vi "Create_Colored_Boolean_Constant.vi"() -> ()   [LabVIEW 2012]
uses:
  <vilib>/Utility/miscctls.llb/LVPointTypeDef.ctl
panel:
  in  "Colors [1]":cluster{"FG Color":u32, "BG Color":u32}[](array[cluster])=[{"FG Color"=42620, "BG Color"=10354663}]
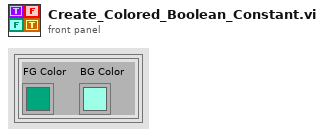
[diagram p1: front panel]
types:
  T1 = typedef "LVPointTypeDef.ctl" = cluster{"Horizontal":i16, "Vertical":i16}
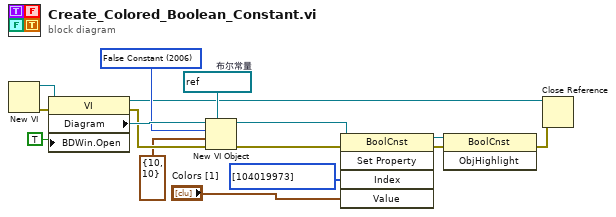
[diagram p0: block diagram]
diagram:
  w5 = u32[] [104019973] items=["Abort Callback"=104256525, "Active Bus"=518639625, "Active Cell:Active Cell"=104038415, "Active Cell:Active Cell"=416911374, "Active Cell:Active Cell"=1955905554, "Active Cell:Active Column Number"=1969896467, "Active Cell:Background Color"=1969896468, "Active Cell:Cell Background Color"=104038417, "Active Cell:Cell Background Color"=416911376, "Active Cell:Cell Background Color"=1955905556, "Active Cell:Cell Font"=104038438, "Active Cell:Cell Font"=416911397, "Active Cell:Cell Font"=1969896500, "Active Cell:Cell Font:Bold"=104038441, "Active Cell:Cell Font:Bold"=416911400, "Active Cell:Cell Font:Bold"=1969896503, "Active Cell:Cell Font:Color"=104038445, "Active Cell:Cell Font:Color"=416911404, "Active Cell:Cell Font:Color"=1969896507, "Active Cell:Cell Font:Italic"=104038442, "Active Cell:Cell Font:Italic"=416911401, "Active Cell:Cell Font:Italic"=1969896504, "Active Cell:Cell Font:Name"=104038439, "Active Cell:Cell Font:Name"=416911398, "Active Cell:Cell Font:Name"=1969896501, "Active Cell:Cell Font:Size"=104038440, "Active Cell:Cell Font:Size"=416911399, "Active Cell:Cell Font:Size"=1969896502, "Active Cell:Cell Font:Strikeout"=104038444, "Active Cell:Cell Font:Strikeout"=416911403, "Active Cell:Cell Font:Strikeout"=1969896506, "Active Cell:Cell Font:Underline"=104038443, "Active Cell:Cell Font:Underline"=416911402, "Active Cell:Cell Font:Underline"=1969896505, "Active Cell:Cell Foreground Color"=1955905555, "Active Cell:Cell Justification"=104038446, "Active Cell:Cell Justification"=416911405, "Active Cell:Foreground Color"=1969896469, "Active Cell:Cell Justification"=1969896508, "Active Cell:Cell Position"=1955905564, "Active Cell:Cell Position:Left"=1955905565, "Active Cell:Cell Position:Top"=1955905566, "Active Cell:Cell Size"=104038418, "Active Cell:Cell Size"=416911377, "Active Cell:Cell Size"=1969896470, "Active Cell:Cell Size:Height"=104038420, "Active Cell:Cell Size:Height"=416911379, "Active Cell:Cell Size:Height"=1969896471, "Active Cell:Cell Size:Width"=104038419, "Active Cell:Cell Size:Width"=416911378, "Active Cell:Cell Size:Width"=1969896472, "Active Cell:Old Cell Size"=1969896485, "Active Cell:OldHeight"=1969896486, "Active Cell:OldWidth"=1969896487, "Active Cell:Position"=104038435, "Active Cell:Position"=416911394, "Active Cell:Position"=1969896497, "Active Cell:Position:Left"=104038436, "Active Cell:Position:Left"=416911395, "Active Cell:Position:Left"=1969896498, "Active Cell:Position:Top"=104038437, "Active Cell:Position:Top"=416911396, "Active Cell:Position:Top"=1969896499, "Active Cell:String"=1969896473, "Active Cursor"=104084485, "Active Cursor"=104090629, "Active Cursor"=960400388, "Active Frame"=1721492482, "Active Item:Child-Only?"=1969896464, "Active Item:Disabled?"=1969896463, "Active Item:Indent Level"=1969896465, "Active Item:Open?"=1969896462, "Active Item:Row Number"=1969896514, "Active Item:Symbol Index"=1969896466, "Active Item:Tag"=1969896461, "Active Plot"=104081412, "Active Plot"=104084483, "Active Plot"=960400386, "Active Plot Area"=960400400, "Active Row:Active Row Number"=104035369, "Active Row:Active Row Position"=104035371, "Active Row:Active Row Position:Left"=104035372, "Active Row:Active Row Position:Top"=104035373, "Active Row:Cell Background Color"=104035374, "Active Row:Cell Font"=104035350, "Active Row:Cell Font:Bold"=104035353, "Active Row:Cell Font:Color"=104035357, "Active Row:Cell Font:Italic"=104035354, "Active Row:Cell Font:Name"=104035351, "Active Row:Cell Font:Size"=104035352, "Active Row:Cell Font:Strikeout"=104035356, "Active Row:Cell Font:Underline"=104035355, "Active Row:Cell Height"=104035370, "Active Row:Cell Justification"=104035358, "Active Slider"=104069123, "Active X Scale"=104078352, "Active Y Scale"=104078353, "Adapt To Entered Data"=98368525, "Adapt To Source"=104050718, "additionalSimulationPrivateData"=126922754, "All Objects []"=104290308, "All Objects[]"=104102916, "All Objects[]"=104105987, "All Supported Methods"=104268801, "All Supported Methods"=104268813, "All Supported Properties"=104265729, "All Supported Properties"=104265742, "All Tags"=1969896515, "Allow Absolute?"=1440002061, "Allow Create New"=49544202, "Allow Create New"=2026532874, "Allow Direct?"=1440002062, "Allow Drag"=103989253, "Allow Dragging"=104093715, "Allow Dragging (Deprecated)"=104035359, "Allow Dropping"=104032277, "Allow Dropping"=104093716, "Allow Editing Cells"=104035360, "Allow Editing Cells"=416911407, "Allow Editing Cells"=1969896509, "Allow Mixed"=867147777, "Allow Multiple Colors"=618574860, "Allow Multiple Names"=49544192, "Allow Multiple Names"=2026532864, "Allow Multiple Names"=3614191617, "Allow Multiple Rows"=618574850, "Allow No Selection"=1475095552, "Allow Preallocation"=104256517, "Allow Read?"=1440002058, "Allow Relative?"=1440002060, "Allow Scanned?"=1440002063, "Allow Selection of Parent Items"=1969896478, "Allow Transparent"=104016900, "Allow Undef Values?"=104130564, "Allow Undefined Names"=49544193, "Allow Undefined Names"=2026532865, "Allow Undefined Names"=3614191616, "Allow Undefined Names"=3813978112, "Allow Undefined Names"=3866933248, "Allow Undefined Strings"=104099842, "Allow Undefined Values"=104062976, "Allow Unwired Left Terminal"=104250373, "Allow User to Open Diagram"=1918386184, "Allow Write?"=1440002059, "AllowCreateNew"=104096791, "AllowCreateNew"=2089216013, "AllowMultiple"=104096780, "AllowMultiple"=2089216008, "AllowObjectDragAndDrop"=1918386190, "AllowRTEdits"=1918386187, "AllowUndefined"=104096779, "AllowUndefined"=2089216007, "Analog Trigger:Show AI Channels"=49544210, "Analog Trigger:Show AI Channels"=2026532882, "Analog Trigger:Show Dedicated"=49544209, "Analog Trigger:Show Dedicated"=2026532881, "Annotation List"=104084508, "Annotation List"=104090638, "Annotation List"=960400402, "Old Annotation List"=104084505, "Old Annotation List"=104090636, "Old Annotation List"=960400391, "Any Thread?"=104256515, "Array Element"=104041479, "Array Input Terminal"=104244227, "Auto Grow?"=618574861, "Auto Sizing"=104102920, "Auto Sizing Style"=104139778, "Auto Sizing?"=104139776, "Automatic Projection Mode"=1358066693, "Autoscale Delay"=104078362, "AutoSize To Fit Contents?"=104204288, "AutoSize To Fit Contents?"=897104897, "Autosizing Row Height"=104035368, "Autosizing Row Height"=104038422, "Autosizing Row Height"=416911381, "Autosizing Row Height"=1969896454, "Auto-Update From Typedef"=104013852, "Auto-Update From Typedef"=104115207, "Available Elements[]"=104250370, "Available Elements[]"=2129913858, "Background Color"=1358066689, "Bad Sub VI Linkage"=104195083, "Bar Plot Style"=103986183, "Basic Object Flags"=103983116, "Bit Accurate Data Size"=104013853, "Blinking"=104013827, "Boolean Text"=104019974, "Bounds"=103983107, "Bounds:Area Height"=103983109, "Bounds:Area Width"=103983108, "Breakpoint Status"=104173580, "Breakpoint Status"=104290314, "Breakpoint Status"=897104905, "Breakpoint?"=104271872, "BreakPoint?"=104271879, "Breakpoint?"=104290310, "Browse Button Rect"=104032276, "Browse Button:Disabled"=104032268, "Browse Button:Visible"=104032267, "Browse Dialog Options"=104032262, "Browse Options"=104032278, "Browse Options:Button Text"=104032275, "Browse Options:Match Pattern"=104032264, "Browse Options:Pattern Label"=104032269, "Browse Options:Prompt"=104032263, "Browse Options:Selection Mode"=104032265, "Browse Options:Start Path"=104032266, "Bus"=518639628, "Bus Open"=518639627, "Button Bar Visible"=104109058, "Button Size"=104019969, "Button Size"=867147778, "Button Size:Height"=104019971, "Button Size:Height"=867147780, "Button Size:Width"=104019970, "Button Size:Width"=867147779, "C Type"=104013862, "Calling Convention"=104256514, "Camera Controller:Auto Redraw"=1358066700, "Camera Controller:Type"=1358066692, "Caption"=104013828, "Caption"=104112133, "Cartesian Lines:Visible"=766554115, "Case Insensitive Match"=104222723, "Case Sensitive Pop-up"=104099846, "Cell FG Color"=104038416, "Cell FG Color"=416911375, "Cell Font"=1955905567, "Cell Font:Bold"=1955905570, "Cell Font:Color"=1955905574, "Cell Font:Italic"=1955905571, "Cell Font:Name"=1955905568, "Cell Font:Size"=1955905569, "Cell Font:Strikeout"=1955905573, "Cell Font:Underline"=1955905572, "Channel:Signal Type"=49544207, "Channel:Signal Type"=2026532879, "Chunk Size Tunnel"=104210440, "Class"=104262656, "Class ID"=103970816, "Class Name"=103970819, "Class Name"=1450114050, "Clump Num"=104173572, "Cluster Size"=104102917, "Cluster Size"=104231936, "Cluster Size:Height"=104102919, "Cluster Size:Width"=104102918, "Code Resource Path"=104253440, "CodeGenMask"=862772224, "Coerce Maximum Value"=1727315973, "Coerce Minimum Value"=1727315972, "Coercion Dot?"=104112134, "Color"=104102913, "Color"=104105984, "Color"=104290304, "Color Area Size"=104016897, "Color Area Size"=104066049, "Color Area Size:Height"=104016899, "Color Area Size:Height"=104066051, "Color Area Size:Width"=104016898, "Color Area Size:Width"=104066050, "Color Table"=104087556, "Color Table"=104090628, "Colors"=103992323, "Colors"=402934794, "Colors"=618574857, "Colors"=2056308738, "Colors [2]"=823938053, "Colors [4]"=104019973, "Colors:BG Color"=103992325, "Colors:BG Color"=402934796, "Colors:BG Color"=618574859, "Colors:BG Color"=2056308740, "Colors:FG Color"=103992324, "Colors:FG Color"=402934795, "Colors:FG Color"=618574858, "Colors:FG Color"=2056308739, "Column Header String"=104035364, "Column Header Strings[]"=104038414, "Column Header Strings[]"=416911365, "Column Header Strings[]"=1969896448, "Companion Diagram"=862772225, "Compare Aggregates?"=104179712, "Concatenate Inputs"=104247296, "Conditions"=1721492481, "Configuration Node"=1817132032, "ConfigurationNode"=1526526976, "Connected Wire"=104112128, "Constructor Node Class Name"=1777212416, "Container Bounds"=104047616, "Container Bounds"=1918386179, "Container Bounds:Height"=104047618, "Container Bounds:Height"=1918386181, "Container Bounds:Width"=104047617, "Container Bounds:Width"=1918386180, "Content Bounds"=1358066694, "Content Bounds:Height"=1358066696, "Content Bounds:Width"=1358066695, "Content Position"=1358066697, "Content Position:Horizontal"=1358066698, "Content Position:Vertical"=1358066699, "Content Rect"=104204293, "Content Rect Bounds"=104035347, "Content Rect Bounds"=104038432, "Content Rect Bounds"=416911391, "Content Rect Bounds"=1955905561, "Content Rect Bounds"=1969896494, "Content Rect Bounds:Height"=104035349, "Content Rect Bounds:Height"=104038434, "Content Rect Bounds:Height"=416911393, "Content Rect Bounds:Height"=1955905563, "Content Rect Bounds:Height"=1969896496, "Content Rect Bounds:Width"=104035348, "Content Rect Bounds:Width"=104038433, "Content Rect Bounds:Width"=416911392, "Content Rect Bounds:Width"=1955905562, "Content Rect Bounds:Width"=1969896495, "Content Rect Position"=104035344, "Content Rect Position"=104038429, "Content Rect Position"=416911388, "Content Rect Position"=1955905558, "Content Rect Position"=1969896491, "Content Rect Position:Left"=104035345, "Content Rect Position:Left"=104038430, "Content Rect Position:Left"=416911389, "Content Rect Position:Left"=1955905559, "Content Rect Position:Left"=1969896492, "Content Rect Position:Top"=104035346, "Content Rect Position:Top"=104038431, "Content Rect Position:Top"=416911390, "Content Rect Position:Top"=1955905560, "Content Rect Position:Top"=1969896493, "Content Rects[]"=897104898, "Control"=104148992, "Control"=104158211, "Control Name"=104155138, "Control Name"=104158208, "Control Reference Linked To"=59413504, "Control Reference Nodes[]"=104013833, "Control Verbs"=104047619, "Controls on Page[]"=402934786, "Controls[]"=104102914, "Controls[]"=104105985, "Convert 4.x data?"=104182784, "Convert 4.x data?"=104185856, "Convert 4.x data?"=104188928, "Cursor"=104044549, "Cursor"=104084486, "Cursor"=104090630, "Cursor"=960400389, "Cursor Color"=103989249, "Cursor Index"=103989256, "Cursor Info"=103989261, "Cursor Legend Visible"=104084496, "Cursor Legend Visible"=104090634, "Cursor Legend Visible"=960400393, "Cursor List"=104084487, "Cursor List"=104084507, "Cursor List"=104090631, "Cursor List"=104090639, "Cursor List"=960400401, "Old Cursor List"=104084506, "Old Cursor List"=104090637, "Old Cursor List"=960400390, "Cursor Lock Style"=103989254, "Cursor Name"=103989248, "Cursor Name Visible"=103989252, "Cursor Plot"=103989255, "Cursor Point Style"=103989251, "Cursor Position"=103989257, "Cursor Position:Cursor X"=103989258, "Cursor Position:Cursor Y"=103989259, "Cursor Style"=103989250, "Custom Rule"=1440002051, "Darken Compare Data"=518639616, "Data Binding:Binding Type"=104013869, "Data Binding:Blink On Alarm"=104013870, "Data Binding:LED Visible"=104013867, "Data Binding:Mode"=104013865, "Data Binding:Path"=104013864, "Data Binding:Persist ID"=104013868, "Data Binding:Status"=104013866, "Data Entry Limits"=46639105, "Data Entry Limits"=104050692, "Data Entry Limits:Increment"=46639108, "Data Entry Limits:Increment"=104050695, "Data Entry Limits:Maximum"=46639107, "Data Entry Limits:Maximum"=104050694, "Data Entry Limits:Minimum"=46639106, "Data Entry Limits:Minimum"=104050693, "Data Offset"=104271881, "DataSocket:Enabled"=104013847, "DataSocket:LED Visible"=104013854, "DataSocket:Mode"=104013846, "DataSocket:Status"=104013848, "DataSocket:URL"=104013845, "Decal Scaling?"=104019980, "DecomposerList[]"=1703848960, "Decorations"=104105986, "Decorations"=104290307, "Decorations on Page[]"=402934787, "Decorations[]"=104102915, "Decrement Key Binding"=104050705, "Default Case"=104222721, "Default Frame"=1721492480, "Default Value"=104013838, "Default Value"=104016901, "Default Value"=104032257, "Default Value"=104038421, "Default Value"=104044548, "Default Value"=104093705, "Default Value"=104096784, "Default Value"=104099841, "Default Value"=1955905537, "Default Value"=3614191619, "Default Value"=3813978114, "Default Value"=3866933250, "Defer Diagram Updates"=104109062, "Defer Panel Updates"=104105989, "Delay"=2005849094, "Deprecated_Flags"=104268806, "Deprecated_Flags[]"=104265735, "Description"=104013839, "Description"=104115201, "Description"=104173570, "Description"=104271874, "Description"=402934791, "Description"=897104900, "Device"=49544199, "Device"=2026532871, "Device String"=104096774, "Device String"=2089216002, "Diagram"=104112130, "Diagram"=104207361, "Diagram Inserted"=1918386189, "Diagrams[]"=104204291, "Diagrams[]"=897104896, "Digital Display"=104056838, "Digital Display"=104066052, "Digital Display"=104127488, "Digital Display(s) Visible"=104081417, "Digital Display[]"=104081411, "Digital Displays[]"=104069131, "Digital Line Style"=103986192, "Digital Transition Location"=103986191, "Digital Transition Type"=103986190, "Digital Tree View"=518639623, "Dimension Sizes"=104041481, "Dimension Sizes"=104121353, "Direction"=2005849088, "Disabled"=104013825, "Disabled"=104013885, "Disabled Items"=104035339, "Disabled Items"=416911362, "Disabled Items []"=104056840, "Disconnect Implicit Enable Signal"=2005849099, "Display Format"=104053766, "Display Format"=104124417, "Display Format Visible?"=104093717, "Display Format Visible?"=104136709, "Display Format:Format"=104053767, "Display Format:Format"=104124418, "Display Format:Precision"=104053768, "Display Format:Precision"=104124419, "Display Style"=104093701, "Display Style"=104136706, "Displayed Items"=1969896476, "DisplayFilter"=104096778, "DisplayFilter"=2089216006, "Doc Max"=1727315969, "Doc Min"=1727315968, "Document Bounds"=103995410, "Document Bounds:Height"=103995412, "Document Bounds:Width"=103995411, "Double-Click"=104035336, "Drag/Drop:Allow Drag and Drop Outside Control"=104035379, "Drag/Drop:Allow Drag and Drop Outside Control"=416911418, "Drag/Drop:Allow Drag and Drop Outside Control"=1969896522, "Drag/Drop:Allow Dragging"=104035376, "Drag/Drop:Allow Dragging"=416911415, "Drag/Drop:Allow Dragging"=1969896518, "Drag/Drop:Allow Dragging (Deprecated)"=416911406, "Drag/Drop:Allow Dragging (Deprecated)"=1969896483, "Drag/Drop:Allow Dragging of Parent Items"=1969896479, "Drag/Drop:Allow Dropping"=104035377, "Drag/Drop:Allow Dropping"=416911416, "Drag/Drop:Allow Dropping"=1969896519, "Drag/Drop:Allow Dropping Between Items"=1969896480, "Drag/Drop:Drag Mode"=104035378, "Drag/Drop:Drag Mode"=416911417, "Drag/Drop:Drag Mode"=1969896521, "Draw Area Size"=104044545, "Draw Companion Diagram Mask"=862772226, "DropDownList[]"=104096781, "DropDownList[]"=2089216009, "Dynamic Library?"=104256522, "Dynamic Parallel Instances Tunnel"=104210438, "Edit Position"=104038409, "Edit Position"=104038449, "Edit Position"=416911420, "Edit Position"=1955905575, "Edit Position"=1969896524, "Old Edit Position"=416911408, "Old Edit Position"=1955905547, "Old Edit Position"=1969896510, "Edit Row"=104035381, "Old Edit Row"=104035361, "Editable"=104001548, "Element"=104026112, "Element"=104121352, "Element Gap?"=104121345, "Element Names[]"=104250368, "Element Names[]"=2129913856, "Elements[]"=104139777, "Embedded Flat Sequence"=1817132036, "Enable Terminal Shown"=2005849095, "Enable Wrapping"=104093714, "Erase First"=104044546, "Error Checking Level"=104256526, "Execution Highlighted Object"=104109060, "Expand Digital Buses"=104007691, "Expand/Contract Symbol:Show Symbol at Root"=1969896520, "Expand/Contract Symbol:Symbol Type"=1969896484, "Expose Typedefs"=919859200, "FeedthroughMap"=126922755, "Fill Color"=104072194, "Fill Style"=104072193, "Fill To"=103986184, "Fill/Point Color"=103986181, "Filter On Device"=49544194, "Filter On Device"=2026532866, "FilterCriteria"=104096793, "FilterCriteria"=2089216016, "FilterOnDevice"=104096777, "FilterOnDevice"=2089216005, "FilterOnSubTypeClass"=104096776, "FilterOnSubTypeClass"=2089216004, "FilterOnTypeClass"=104096775, "FilterOnTypeClass"=2089216003, "Fire Count"=104173574, "Firing Order"=104290312, "Fix Contents"=104204297, "Fixed Tab Dimension"=618574849, "Fixed Tab Dimension:Height"=618574856, "Fixed Tab Dimension:Width"=618574855, "Fixed-Point Overflow Status Visible?"=98368527, "Fixed-Point Overflow Status Visible?"=104050720, "Fixed-Point Representation:Actual"=98368521, "Fixed-Point Representation:Actual"=104050714, "Fixed-Point Representation:Actual:Delta"=98368524, "Fixed-Point Representation:Actual:Delta"=104050717, "Fixed-Point Representation:Actual:Range Max"=98368523, "Fixed-Point Representation:Actual:Range Max"=104050716, "Fixed-Point Representation:Actual:Range Min"=98368522, "Fixed-Point Representation:Actual:Range Min"=104050715, "Fixed-Point Representation:Bits"=98368513, "Fixed-Point Representation:Bits"=104050706, "Fixed-Point Representation:Bits:Integer Word Length"=98368516, "Fixed-Point Representation:Bits:Integer Word Length"=104050709, "Fixed-Point Representation:Bits:Signed"=98368514, "Fixed-Point Representation:Bits:Signed"=104050707, "Fixed-Point Representation:Bits:Word Length"=98368515, "Fixed-Point Representation:Bits:Word Length"=104050708, "Fixed-Point Representation:Desired"=98368517, "Fixed-Point Representation:Desired"=104050710, "Fixed-Point Representation:Desired:Delta"=98368520, "Fixed-Point Representation:Desired:Delta"=104050713, "Fixed-Point Representation:Desired:Range Max"=98368519, "Fixed-Point Representation:Desired:Range Max"=104050712, "Fixed-Point Representation:Desired:Range Min"=98368518, "Fixed-Point Representation:Desired:Range Min"=104050711, "Fixed-Point Representation:Include Overflow Status?"=98368526, "Fixed-Point Representation:Include Overflow Status?"=104050719, "Flags:Has Deprecated"=104265739, "Flags:Has Ignore Errors Inside Node"=104265744, "Flags:Has Must Run At Root Loop"=104265740, "Flags:Has Not Available In AppLibs"=104265736, "Flags:Has Private"=104265737, "Flags:Has Risky Scripting"=104265741, "Flags:Has Scripting"=104265738, "Flags:Is Deprecated"=104268810, "Flags:Is Private"=104268808, "Flags:Is Risky Scripting"=104268812, "Flags:Is Scripting"=104268809, "Flags:Must Run At Root Loop"=104268811, "Flags:Not Available In AppLibs"=104268807, "Flange 1:Depth"=823938050, "Flange 1:Width"=823938048, "Flange 2:Depth"=823938051, "Flange 2:Width"=823938049, "Flavor"=104062982, "Flavor"=104130563, "Flipped"=104001546, "Focus Key Binding"=104013840, "Font"=103995393, "Font:Bold"=103995401, "Font:Color"=103995405, "Font:Italic"=103995402, "Font:Name"=103995399, "Font:Size"=103995400, "Font:Strikeout"=103995404, "Font:Underline"=103995403, "FontType"=103995416, "Force Unicode Text"=104093706, "Format"=1955905545, "Format & Precision"=103998464, "Format & Precision"=104001537, "Format & Precision:Format"=103998465, "Format & Precision:Format"=104001538, "Format & Precision:Precision"=103998466, "Format & Precision:Precision"=104001539, "Format String"=46639104, "Format String"=103998467, "Format String"=104001558, "Format String"=104053765, "Format String"=104124422, "Format String"=104259584, "Format String"=1090016256, "Formula Expression"=104225793, "Formula Parameters[]"=104225794, "Frame Count"=104216579, "Frame Names"=104222722, "Frame Rectangle"=104204294, "Frame Selector Rect"=104216578, "Frame Size"=104204290, "Frames[]"=104216577, "Frames[]"=897104903, "Full Element Index[]"=104250372, "Full Element Index[]"=2129913860, "Full Element Names[]"=104250371, "Full Element Names[]"=2129913859, "Full Name"=890692608, "Full Names Visible?"=104250369, "Full Names Visible?"=2129913857, "Function Name"=104256513, "Functions[]"=104290305, "Genericity"=104013884, "GetVRTILOErrors"=1440002066, "Graph Flavor"=104078357, "Grayed When VI Reserved"=104096797, "Grid Colors"=104007687, "Grid Colors"=104078344, "Grid Colors:Major Color"=104007688, "Grid Colors:Minor Color"=104007689, "Grid Colors:X Color"=104078345, "Grid Colors:Y Color"=104078346, "Group Member Refs[]"=103983112, "Grouped"=103983110, "Grow Info"=104013871, "Grow Info:Can Grow Horizontally"=104013872, "Grow Info:Can Grow Vertically"=104013873, "Grow Info:Max Horizontally"=104013876, "Grow Info:Max Vertically"=104013877, "Grow Info:Min Horizontally"=104013874, "Grow Info:Min Vertically"=104013875, "Grow Terms"=104195074, "GUID"=890692609, "Has Caption"=104013858, "Has Conditional Terminal?"=104210433, "Has Side Effects?"=104176642, "Has Sub-Diagram"=890692611, "Header Appearance"=2005849097, "Hide Last Value"=104056852, "Hide Text"=46639114, "Hide Text"=104053769, "High Color"=104004610, "High Color"=104010759, "Highlight Execution?"=104109059, "Horizontal Scrollbar Visible"=104041483, "Horizontal Scrollbar Visible"=104044556, "Horizontal Scrollbar Visible"=104093713, "Horizontal Scrollbar Visible"=104121356, "Horizontal Scrollbar Visible"=104139780, "Horizontal Scrollbar Visible"=1955905542, "Housing Colors"=104069133, "Housing Colors:BG Color"=104069135, "Housing Colors:FG Color"=104069134, "Housing Length"=1727315975, "Housing Size"=104069120, "Housing Size:Height"=104069122, "Housing Size:Width"=104069121, "Icon"=104173576, "Ignore Array"=104087555, "Ignore Array"=104090627, "Ignore Attributes"=104081427, "Ignore Attributes"=104084499, "Ignore Attributes"=960400395, "Ignore Errors Inside Node?"=104265733, "Ignore FPGA Reset Method"=2005849098, "Ignore Separators"=104096798, "Ignore Separators"=2089216019, "Ignore Timestamp"=104084498, "Ignore Timestamp"=960400394, "Include Invalid Names"=49544201, "Include Invalid Names"=2026532873, "Include Lower Limit?"=8582144, "Include Upper Limit?"=8582145, "IncludeInvalid"=104096790, "IncludeInvalid"=2089216012, "Increment"=1727315970, "Increment Key Binding"=104050704, "Increment/Decrement Visible?"=104053764, "Increment/Decrement Visible?"=104056851, "Independent Label"=402934793, "Index Count"=104244224, "Index Mode"=104164352, "Index Rect"=104041484, "Index Rect"=104121357, "Index Terminals[][]"=104244225, "Index Value"=104121349, "Index Values"=104038410, "Index Values"=104041476, "Index Visible"=104041475, "Index Visible?"=104121348, "Indicator"=104013831, "Initialization Type"=2005849096, "Initializer Is On Loop"=2005849093, "Initializer Terminal"=2005849091, "Initializer's Loop"=2005849092, "Input Count"=1460327424, "Input Terminal"=2005849090, "Input Terminals"=1460327425, "Input Terminals []"=104268804, "Input Terminals []"=1777212417, "Input Terminals[]"=104253442, "Input Terminals[]"=104256520, "Input?"=104152065, "Inside Terminals[]"=104161280, "Interpolate Color"=104004608, "Interpolate Color"=104010757, "Interpret As Unicode"=103995409, "Invert Inputs?[]"=104241153, "Invoke Node Class Name"=104268802, "Invoke Nodes[]"=104013836, "IOVLocalAccessMode"=1440002064, "Is Array?"=104035365, "Is Array?"=416911411, "Is Array?"=1969896513, "Is Asynchronous"=104173575, "Is Break Point Set"=104173571, "Is Break Point Set"=897104902, "Is Broken?"=104271876, "Is Debugging Allowed"=104210439, "Is On Block Diagram?"=103970821, "Is On Connector Pane"=104013856, "Is Parallelism Enabled?"=104210436, "Is Private Class Selected"=1450114052, "Is Run At Any Loop"=104173578, "Is Scripting Class Selected"=1450114051, "Is Source?"=104112131, "Is Strict"=1280954370, "Is Strict?"=1771824128, "Is Stub?"=104013883, "Is Typedef?"=104013850, "Is Typedef?"=104115205, "Is Vertical?"=2056308736, "Is Wizard Locked"=103983117, "IsCompilation"=862772227, "IsTracking"=104019977, "Item Names"=104035337, "Item Names"=416911360, "Item Symbols"=104035338, "Item Symbols"=416911361, "Items[]"=104127489, "Joints[]"=104271877, "Justification"=103995413, "Justify Tabs"=618574851, "Key Focus"=104013826, "Keyboard Mode"=104035332, "Keyboard Mode"=416911412, "Keyboard Mode"=1969896459, "Label"=104013829, "Label"=104115202, "Label"=104148993, "Label"=104155139, "Label"=104158210, "Label"=104173569, "Label"=897104899, "Label"=2056308743, "Label Format"=103986189, "Latch Value"=104013855, "Left Data Node"=1526526981, "Left Registers[]"=104167424, "Legend:Autosize"=104081425, "Legend:Autosize"=104084500, "Legend:Disable"=104081426, "Legend:Disable"=104084501, "Legend:Disable"=960400396, "Legend:Number of Rows"=104081428, "Legend:Number of Rows"=104084510, "Legend:Plot Minimum"=104081429, "Legend:Plot Minimum"=104084509, "Legend:Plots Shown"=104081424, "Legend:Plots Shown"=104084495, "Legend:Position"=104081418, "Legend:Position"=104084489, "Legend:Position:Left"=104081419, "Legend:Position:Left"=104084490, "Legend:Position:Top"=104081420, "Legend:Position:Top"=104084491, "Legend:Scrollbar Visible"=104081430, "Legend:Scrollbar Visible"=104084511, "Legend:Size"=104081421, "Legend:Size"=104084492, "Legend:Size:Height"=104081423, "Legend:Size:Height"=104084494, "Legend:Size:Width"=104081422, "Legend:Size:Width"=104084493, "Legend:Visible"=104081409, "Legend:Visible"=104084481, "Legend:Visible"=960400384, "Library Path"=104256512, "Limit To Single Line?"=104093703, "Limit To Single Line?"=104136707, "Line Style"=103986180, "Line Style"=103989262, "Line Width"=103986182, "Line Width"=103989263, "Linked Control"=104265734, "Linked Control"=104268803, "Load and Retain"=104198146, "Local Variables[]"=104013834, "Lock"=103995415, "Lock"=104075265, "Lock Boolean Text In Center"=104019975, "Locked"=103983111, "Loop Count"=104210432, "Loop Counter"=104207360, "Loop End Ref"=104210434, "Loop End Ref"=104213504, "Loose Fit"=104007684, "Loose Fit"=104010756, "Low Color"=104004609, "Low Color"=104010758, "Mapping Mode"=104001547, "Marker"=104001557, "Marker Colors"=104001554, "Marker Colors:BG Color"=104001556, "Marker Colors:Text Color"=104001555, "Marker Values[]"=104004611, "Marker Values[]"=104007685, "Marker Values[]"=104010760, "Master Bounds Rect"=103983115, "MatchFirstInList"=104099847, "Mechanical Action"=104019976, "Mechanical Action"=1475095553, "Menu Button Visible"=104096795, "Menu Button Visible"=2089216018, "Menubar Visible"=104105993, "Menubar Visible"=104109057, "Method"=104268800, "Method"=104268814, "Minor Tick Color"=104001550, "Mode"=104241152, "ModelView Matrix"=1358066688, "Modified"=103970820, "Mouse"=104044547, "Multiple Line Input"=104035367, "Multiple Line Input"=104038424, "Multiple Line Input"=416911383, "Multiple Line Input"=1969896455, "Multiple Text String"=104019978, "Name"=104112132, "Name"=104152064, "Name Format"=104262657, "Name Label"=104007686, "Name Label"=104010762, "Named Numeric Colors"=104056835, "Named Numeric Colors:BG Color"=104056837, "Named Numeric Colors:Text Color"=104056836, "Named Numeric Font"=104056842, "Named Numeric Font:Bold"=104056845, "Named Numeric Font:Color"=104056849, "Named Numeric Font:Italic"=104056846, "Named Numeric Font:Name"=104056843, "Named Numeric Font:Size"=104056844, "Named Numeric Font:Strikeout"=104056848, "Named Numeric Font:Underline"=104056847, "Named Numeric Size"=104056832, "Named Numeric Size:Height"=104056834, "Named Numeric Size:Width"=104056833, "NI Validated"=104256518, "Nodes"=104290313, "Num Dimensions"=104121344, "Num Of Sliders"=104069128, "Number of Columns"=104038401, "Number of Columns"=104041473, "Number of Columns"=104121346, "Number of Columns"=416911370, "Number of Columns"=1969896452, "Number Of Dimensions"=104041480, "Number of Items"=104056841, "Number of Rows"=104035329, "Number of Rows"=104038402, "Number of Rows"=104041474, "Number of Rows"=104121347, "Number of Rows"=416911369, "Number of Rows"=1969896451, "Number of Static Parallel Instances"=104210437, "Numeric Text"=46639113, "Numeric Text"=104053763, "Numeric Text"=104124423, "Numeric Text"=1090016257, "Objects on Page[]"=402934788, "Offset and Multiplier"=104007681, "Offset and Multiplier"=104010753, "Offset and Multiplier:Multiplier"=104007683, "Offset and Multiplier:Multiplier"=104010755, "Offset and Multiplier:Offset"=104007682, "Offset and Multiplier:Offset"=104010754, "Old Cursor List"=104084497, "Old Format & Precision"=104050688, "Old Format & Precision:Old Format"=104050689, "Old Format & Precision:Old Precision"=104050690, "Old Format String"=104050703, "Old Out of Range Action"=104050696, "Old Range"=104001553, "Optional Plane:Labels Visible"=766554114, "Optional Plane:Lines Visible"=766554113, "Optional Plane:Plane Type"=766554112, "Origin"=104044550, "Origin"=1918386188, "Origin:Left"=104044551, "Origin:Left"=404044551, "Origin:Top"=104044552, "Output Count"=1556456448, "Output Node"=1817132033, "Output Terminal"=2005849089, "Output Terminals []"=104256519, "Output Terminals []"=104268805, "Output Terminals []"=1777212418, "Output Terminals[]"=104244228, "Output Terminals[]"=104253443, "Output Terminals[]"=1556456449, "Output Terminals[] (Deprecated)"=104244226, "OutputNode"=1526526977, "Outside Terminal"=104161281, "Owner (Deprecated)"=103970817, "Owner"=103970822, "Owning VI"=103970818, "Page Enabled State"=402934784, "Page Label"=402934790, "Page Labels Display Visible?"=618574863, "Page Selector Visible"=65605632, "Page Size"=1727315971, "Page Visible"=402934785, "Pages"=65605633, "Palette:Active Tool"=104078351, "Palette:Visible"=104078339, "Panel Transparent"=1918386178, "Panes"=104105990, "Parallel Schedule"=104210441, "Parameter Info"=104256516, "Parameter Info"=104256521, "ParameterCount"=104253441, "Path Text"=104032261, "Path Type"=104118274, "Physical Channel:Show External"=49544216, "Physical Channel:Show External"=2026532888, "Physical Channel:Show Internal"=49544217, "Physical Channel:Show Internal"=2026532889, "Physical Channel:Show Internal Bizarre"=49544218, "Physical Channel:Show Internal Bizarre"=2026532890, "Physical Channel:Signal Type"=49544208, "Physical Channel:Signal Type"=2026532880, "Pipe Radius"=823938052, "Pixel Width"=104035330, "Plot"=104081413, "Plot"=104084484, "Plot"=960400387, "Plot Area Bounds"=104078361, "Plot Area:Colors"=104078341, "Plot Area:Colors:BG Color"=104078343, "Plot Area:Colors:FG Color"=104078342, "Plot Area:Position"=104078358, "Plot Area:Position:Left"=104078359, "Plot Area:Position:Top"=104078360, "Plot Area:Size"=104078336, "Plot Area:Size:Height"=104078338, "Plot Area:Size:Width"=104078337, "Plot Color"=103986177, "Plot Images:Back"=104084502, "Plot Images:Back"=960400397, "Plot Images:Front"=104084504, "Plot Images:Front"=104090635, "Plot Images:Front"=960400399, "Plot Images:Middle"=104084503, "Plot Images:Middle"=960400398, "Plot Info"=103986188, "Plot Interpolation"=103986178, "Plot Name"=103986176, "Point Style"=103986179, "Position"=103983104, "Position:Left"=103983105, "Position:Top"=103983106, "Prealloc Length"=104093707, "Prealloc Length"=104136708, "Probe"=104271873, "ProbeVI"=104274945, "Projection Matrix"=1358066691, "Properties[]"=104265728, "Properties[]"=104265743, "Property Count"=104265731, "Property Items[]"=104265730, "Property Node Class Name"=104265732, "Property Nodes[]"=104013835, "Radix Visible?"=104053762, "Radix Visible?"=104124420, "Ramp Visible"=104004612, "Ramp Visible"=104010761, "Range"=104001540, "Range:Increment"=104001543, "Range:Maximum"=104001542, "Range:Minimum"=104001541, "Range:Minor Increment"=104001544, "Range:Start"=104001545, "Recomposer List[]"=1703848961, "Region Nodes[]"=890692610, "Relative Mode"=1440002052, "Reload For Each Call"=104198145, "Representation"=98368512, "Representation"=104050691, "Representation"=1727315974, "Reserve Callback"=104256523, "Resize Info:Can Resize Horizontally"=103983119, "Resize Info:Can Resize Vertically"=103983120, "Resize Info:Include In Resize"=103983122, "Resize Info:Name in Resize Dialog"=103983121, "Resource Id"=104176643, "Response to Value Outside Limits"=46639109, "Response to Value Outside Limits"=104050699, "Response to Value Outside Limits:Increment"=46639112, "Response to Value Outside Limits:Increment"=104050702, "Response to Value Outside Limits:Maximum"=46639110, "Response to Value Outside Limits:Maximum"=104050700, "Response to Value Outside Limits:Minimum"=46639111, "Response to Value Outside Limits:Minimum"=104050701, "RestrictLRGrowMove"=104250374, "RestrictLRGrowMove"=2129913861, "RGB Value"=104066055, "Right Data Node"=1526526982, "Right Shift Register"=104287232, "Ring Text"=104056850, "Row Header Strings[]"=104038413, "Row Header Strings[]"=416911410, "Row Header Strings[]"=1969896512, "Scale"=104066053, "Scale"=104072195, "Scale"=104075264, "Scale Fit"=104007680, "Scale Fit"=104010752, "Scale Info"=104066054, "Scale Info"=104069132, "Scale Legend:Visible"=104078354, "Scale Panel"=1918386176, "Scroll Position"=103995397, "Scrollbar Visible"=104032274, "Scrollbar Visible"=104093702, "Scrollbar Visible?"=104118273, "Scrollbar Visible?"=104136705, "Scrollbar Visible?"=104225792, "Scrollbars Visible"=104044554, "Select Entire Rows"=104035380, "Select Entire Rows"=416911419, "Select Entire Rows"=1969896523, "Selected"=103983113, "Selected Cell"=416911384, "Selected Cursors"=104084488, "Selected Cursors"=104090632, "Selected Cursors"=960400392, "Selection"=103995394, "Selection Color"=104035366, "Selection Color"=104038408, "Selection Color"=416911380, "Selection Color"=1955905550, "Selection Color"=1969896456, "Selection End[]"=104121351, "Selection List[]"=104105988, "Selection List[]"=104109056, "Selection Mode"=104035331, "Selection Mode"=416911373, "Selection Mode"=1969896460, "Selection Size"=104038412, "Selection Size"=1955905549, "Selection Size[]"=104041478, "Selection Start"=104038411, "Selection Start"=1955905548, "Selection Start[]"=104041477, "Selection Start[]"=104121350, "Selection:End"=103995396, "Selection:Start"=103995395, "SelectionModeFlags"=289982464, "Selector"=104222720, "Sequence Locals[]"=104219648, "Shared Clones:Automatic Allocation Strategy Enabled"=104204295, "Shared Clones:Pre-Allocate"=104204296, "Shared Variable Project Item"=1440002048, "Shift Registers[]"=104207362, "Short Count"=104173573, "Show Buses With Lines"=518639624, "Show Selection?"=104121354, "Show Timeout?"=1440002053, "Show Timestamp?"=1440002050, "Show Value Tip Strip"=104069136, "Sibling Multiselect"=1969896516, "Signal Numbers Visible"=1955905544, "SimDiagisDirty"=126922756, "SimulationDiagram"=1988411392, "SimulationParameters"=126922753, "Size"=103992320, "Size"=104032271, "Size"=104035341, "Size"=104038426, "Size"=104093709, "Size"=104096786, "Size"=416911385, "Size"=1955905538, "Size"=1969896488, "Size to Text?"=103995398, "Size To Text?"=104118272, "Size To Text?"=104136704, "Size:Height"=103992322, "Size:Height"=104032273, "Size:Height"=104035343, "Size:Height"=104038428, "Size:Height"=104093711, "Size:Height"=104096788, "Size:Height"=416911387, "Size:Height"=1955905540, "Size:Height"=1969896490, "Size:Width"=103992321, "Size:Width"=104032272, "Size:Width"=104035342, "Size:Width"=104038427, "Size:Width"=104093710, "Size:Width"=104096787, "Size:Width"=416911386, "Size:Width"=1955905539, "Size:Width"=1969896489, "Sizing"=2056308742, "Skip Subroutine Call If Busy"=104195077, "Skip When Tabbing"=104013857, "Slider Colors"=104069124, "Slider Colors:BG Color"=104069126, "Slider Colors:FG Color"=104069125, "Smooth Horizontal Scrolling"=104038423, "Smooth Horizontal Scrolling"=416911382, "Smooth Update"=104084482, "Smooth Update"=104090625, "Smooth Update"=960400385, "SnaptoMouse"=104075266, "Source Addressing Mode"=104271880, "Splitter Position"=2056308737, "Splitter Position Locked"=2056308741, "Splitters[]"=104105991, "Stack Plots?"=104081415, "State Nodes[]"=827376640, "Static VI Path"=104198144, "StaticState"=862772228, "Stop If True?"=104210435, "Stop If True?"=104213505, "Strings []"=104056839, "Strings []"=104099843, "Strings []"=867147776, "Strings []"=2145735680, "Strings [4]"=104019972, "Strings And Values []"=104062980, "Strings And Values []"=104099844, "Strings And Values []"=104130561, "Strings And Values []"=2145735681, "Style"=104001536, "Style"=104142848, "Style"=104173577, "Style"=104176641, "Style ID"=104013882, "SubTypeClass"=104096773, "SubTypeClass"=2089216001, "SubVI Setup:Close Front Panel After Call"=104195081, "SubVI Setup:Open Front Panel When Loaded"=104195079, "SubVI Setup:Show Front Panel When Called"=104195080, "SubVI Setup:Suspend When Called"=104195082, "SubVIs[]"=104290306, "Switch:Show Channels"=49544211, "Switch:Show Channels"=2026532883, "Switch:Show Relays"=49544212, "Switch:Show Relays"=2026532884, "Switch:Show Topologies"=49544219, "Switch:Show Topologies"=2026532891, "Synch Current And Default Values"=104096796, "Synchronous Display"=104013832, "Synchronous I/O?"=104192000, "Tab Caption"=402934789, "Tab Control Pane Dimension"=618574852, "Tab Control Pane Dimension:Height"=618574854, "Tab Control Pane Dimension:Width"=618574853, "Tab Into"=618574866, "Tab Layout"=618574864, "Tab Location"=618574865, "Tab Size"=618574848, "Tabs Visible?"=618574862, "TagList[]"=104096789, "TagList[]"=2089216011, "TagType"=49544200, "TagType"=104096783, "TagType"=2026532872, "TagType"=2089216014, "Target Syntax Checking"=104204292, "Target Syntax Checking"=897104904, "Terminal"=104013830, "Terminal"=104115204, "Terminal"=104152066, "Terminal"=1450114049, "Terminal Height"=104235008, "Terminal:Show Advanced"=49544214, "Terminal:Show Advanced"=2026532886, "Terminal:Show Basic"=49544213, "Terminal:Show Basic"=2026532885, "Terminal:Show Private"=49544215, "Terminal:Show Private"=2026532887, "Terminals Visible?"=104176640, "Terminals Visible?"=104195072, "Terminals[]"=104170496, "Terminals[]"=104173568, "Terminals[]"=104271875, "Terminals[]"=897104901, "Text"=103995392, "Text"=104093700, "Text"=104096771, "Text"=867147781, "Text Colors"=103995406, "Text Colors:BG Color"=103995408, "Text Colors:Text Color"=103995407, "Text Focus"=104105992, "Text Focus"=104109061, "Text Labels Visible?"=104069129, "Text Labels[]"=104069130, "Text Size"=104032258, "Text Size"=104093697, "Text Size"=104096768, "Text Size:Height"=104032260, "Text Size:Height"=104093699, "Text Size:Height"=104096770, "Text Size:Width"=104032259, "Text Size:Width"=104093698, "Text Size:Width"=104096769, "Text Width"=104053761, "Tick Color"=104001549, "Timed Loop Left DCO"=1526526978, "Timed Loop Right DCO"=1526526979, "Timed Sequence Left DCO"=1817132034, "Timed Sequence Right DCO"=1817132035, "Timeout Allowed?"=1440002054, "Timestamp Allowed?"=1440002065, "Tip Strip"=104013844, "Tip Strip"=104115203, "Tip Strip"=402934792, "TL Timed Sequence"=1526526980, "Toggle Key Binding"=104019979, "Toggle Key Binding"=867147782, "Top Left Cell"=1955905546, "Top Left Visible Cell"=416911372, "Top Left Visible Cell"=1969896457, "Top Row"=104035335, "Total Bounds Rect"=103983114, "Transitions Visible"=1955905543, "Transpose Array"=104078340, "Tunnel"=104284160, "Tunnels[]"=104204289, "Twisty Type"=1969896474, "Type"=1450114048, "Type Class"=1493837824, "Type Descriptor"=104013841, "Type Descriptor"=104112129, "Type Descriptor (Full)"=104013863, "TypeClass"=104096772, "TypeClass"=2089216000, "Typedef:Path"=104013851, "Typedef:Path"=104115206, "Typedef:VI"=104013861, "Typedef:VI"=104115208, "UID"=103983123, "Uniform Marker Spacing?"=104001551, "Unit"=104201216, "Unit Label"=104007690, "Unit Label"=104010763, "Unit Label"=104050698, "Unit Label"=104124424, "Unit Label Visible?"=104124421, "Unreserve Callback"=104256524, "Update Mode"=104081414, "Update Mode"=104087557, "Update While Typing?"=104093704, "UpdatedTagList[]"=104096792, "UpdatedTagList[]"=2089216015, "User Data"=104023040, "User Data"=104096794, "User Data"=1333814273, "User Data"=2089216017, "Value"=104013837, "Value"=104016896, "Value"=104032256, "Value"=104038400, "Value"=104044544, "Value"=104093696, "Value"=104096782, "Value"=104099840, "Value"=104115200, "Value"=1333814272, "Value"=1918386185, "Value"=1955905536, "Value"=2089216010, "Value"=3614191618, "Value"=3813978113, "Value"=3866933249, "Value (Signaling)"=104013859, "Value (Signaling)"=104016902, "Value (Signaling)"=104032270, "Value (Signaling)"=104038425, "Value (Signaling)"=104044555, "Value (Signaling)"=104093708, "Value (Signaling)"=104096785, "Value (Signaling)"=104099845, "Value (Signaling)"=1918386186, "Value (Signaling)"=1955905557, "Value (Signaling)"=3614191620, "Value (Signaling)"=3813978115, "Value (Signaling)"=3866933251, "Values []"=104062979, "Values []"=104130560, "Vertical Arrangement"=103995414, "Vertical Scrollbar Visible"=104041482, "Vertical Scrollbar Visible"=104044557, "Vertical Scrollbar Visible"=104093712, "Vertical Scrollbar Visible"=104121355, "Vertical Scrollbar Visible"=104139779, "Vertical Scrollbar Visible"=1955905541, "VI Name"=104155136, "VI Name"=104195073, "VI Name"=1280954368, "VI Path"=104195075, "VI Path"=1280954369, "VI Reference"=104195078, "View As Icon"=104139781, "View As Icon"=104195076, "Visible"=103986187, "Visible"=103989260, "Visible"=103992326, "Visible"=104001552, "Visible"=104013824, "Visible"=104173579, "Visible Bounds"=104290311, "Visible Frame"=104216576, "Visible Items:Column Header Visible"=104035363, "Visible Items:Column Headers Visible"=104038407, "Visible Items:Column Headers Visible"=416911371, "Visible Items:Column Headers Visible"=1969896453, "Visible Items:Hierarchy Lines Visible"=1969896525, "Visible Items:Hierarchy Lines Visible Old"=1969896477, "Visible Items:Horizontal Lines Visible"=104035375, "Visible Items:Horizontal Lines Visible"=104038447, "Visible Items:Horizontal Lines Visible"=416911414, "Visible Items:Horizontal Lines Visible"=1969896482, "Visible Items:Horizontal Scrollbar Visible"=104038405, "Visible Items:Horizontal Scrollbar Visible"=416911368, "Visible Items:Horizontal Scrollbar Visible"=1969896450, "Visible Items:Index Visible"=104038403, "Visible Items:Row Headers Visible"=104038406, "Visible Items:Row Headers Visible"=416911409, "Visible Items:Row Headers Visible"=1969896511, "Visible Items:Symbols Visible"=104035334, "Visible Items:Symbols Visible"=416911366, "Visible Items:Symbols Visible"=1969896458, "Visible Items:Vertical Lines Visible"=104038448, "Visible Items:Vertical Lines Visible"=416911413, "Visible Items:Vertical Lines Visible"=1969896481, "Visible Items:Vertical Scrollbar Visible"=104035333, "Visible Items:Vertical Scrollbar Visible"=104038404, "Visible Items:Vertical Scrollbar Visible"=416911367, "Visible Items:Vertical Scrollbar Visible"=1969896449, "Wire"=104274944, "Wire Width"=104271878, "Wires[]"=104290309, "Wizard Data"=104013849, "Write?"=104155137, "Write?"=104158209, "Write?"=1440002049, "X Scale"=104078347, "X Scale Index"=103986185, "X Scale Info"=104078349, "X Scrollbar Visible"=104078356, "X Scrollbar Visible"=1918386182, "XControl:Container Bounds"=104013879, "XControl:Container Bounds:Height"=104013881, "XControl:Container Bounds:Width"=104013880, "XControl:Is XControl?"=104013878, "Y Scale"=104078348, "Y Scale Index"=103986186, "Y Scale Info"=104078350, "Y Scrollbar Visible"=1918386183, "Z Scale"=104087554, "Z Scale"=104090626, "Z Scale Info"=104090633, "Zoom Factor"=104044553] ("Index")
  w9 = refnum<vi> refnum  # 布尔常量
  w11 = 2006 items=[".NET Container"=2125, ".NET Refnum"=3441, "2D Picture"=3508, "3D Picture"=23776, "Absolute Value"=1054, "Access Rights"=1412, "ActiveX Container"=2072, "Add"=1050, "Add (with error terminals)"=3915, "Add Array Elements"=1903, "Agitator"=3831, "AllSpoll"=1960, "Always Copy"=2400, "And"=1061, "And Array Elements"=1911, "Append True/False String"=1511, "Application Refnum"=3412, "Array (block diagram constant)"=2070, "Array (classic)"=3300, "Array (modern)"=21608, "Array Interface Control"=23777, "Array Max & Min"=1907, "Array of Strings to Path"=1422, "Array Size"=1809, "Array Subset"=2044, "Array To Cluster"=1168, "Array To Spreadsheet String"=1540, "Atmospheric Tank (classic)"=3070, "Atmospheric Tank (modern)"=21751, "Automation Close"=8001, "Automation Open"=8000, "Automation Refnum"=3410, "Avogadro Constant (1/mol)"=23520, "Base 10 Logarithm Of e"=23512, "Bin #1"=3073, "Bin #2"=21755, "Bitpack to Array"=3135, "Bluetooth Close Connection"=9148, "Bluetooth Create Listener"=9151, "Bluetooth Discover"=9152, "Bluetooth Network Connection Refnum"=3468, "Bluetooth Open Connection"=9153, "Bluetooth Read"=9149, "Bluetooth Wait On Listener"=9147, "Bluetooth Write"=9150, "Boolean Array To Number"=1815, "Boolean To (0,1)"=1167, "Build Array"=2041, "Build Cluster Array"=2047, "Build Matrix"=8500, "Build Path"=1419, "Build Waveform"=2066, "Bundle"=2049, "Bundle By Name"=2057, "Byte Array To String"=1609, "Byte Stream File Refnum"=3408, "Call By Reference"=3901, "Call Chain"=1999, "Call Library Function Node"=2062, "Call Parent Method"=2354, "CAN Channel (block diagram constant)"=2124, "CAN Channel (classic)"=3340, "CAN Channel (modern)"=21817, "CAN Channel (system)"=21966, "CAN Interface (block diagram constant)"=2123, "CAN Interface (classic)"=3339, "CAN Interface (modern)"=21815, "CAN Interface (system)"=21964, "CAN Task (block diagram constant)"=3471, "CAN Task (classic)"=3470, "CAN Task (modern)"=21789, "CAN Task (system)"=21963, "Cancel Button (modern)"=21739, "Cancel Button (system)"=3131, "Cancel Notification"=9107, "Carriage Return Constant"=23500, "Case Structure"=2001, "Cast Unit Bases"=1079, "Check Valve"=3833, "Checkbox (classic)"=3117, "CheckBox (modern)"=21924, "Checkbox (system)"=3132, "Class Specifier Constant"=2094, "Clear Fixed-Point Overflow Status"=5562, "Close File"=8052, "Close File (deprecated)"=1405, "Close Reference"=8011, "Close Variable Connection"=23783, "Cluster (classic)"=3400, "Cluster (modern)"=21607, "Cluster Constant"=2071, "Cluster To Array"=1169, "Code Interface Node"=2050, "Coerce To Type"=2402, "Color Box"=3013, "Color Box Constant"=2120, "Color Box Thin Border"=2905, "Color Ramp"=3022, "Colored Rectangle (broken?)"=3625, "Combo Box (classic)"=3304, "Combo Box (modern)"=21604, "Combo Box (system)"=21917, "Combo Box Constant"=2088, "Complex Conjugate"=1048, "Complex To Polar"=1045, "Complex To Re/Im"=1044, "Compound Arithmetic"=2200, "Compressor"=3832, "Concatenate Strings"=2040, "Conditional Disable Structure"=2064, "Constructor Node"=3904, "Control & Simulation Loop"=2099, "Control Help Window"=1353, "Control Online Help"=1355, "Control Refnum"=3419, "Convert Unit"=2059, "Conveyer"=3827, "Copy"=8053, "Copy (deprecated)"=1416, "Cosecant"=1204, "Cosine"=1201, "Cotangent"=1205, "CPU Information"=24130, "Create Folder"=8055, "Create Network Stream Reader Endpoint"=23811, "Create Network Stream Writer Endpoint"=23810, "Create Stream"=23796, "Create User Event"=2073, "Current Processor ID"=24131, "Current VI's Menubar"=9000, "Current VI's Path"=1426, "DAQmx Analog Trigger Source (block diagram constant)"=2119, "DAQmx Analog Trigger Source (classic)"=3336, "DAQmx Analog Trigger Source (modern)"=21774, "DAQmx Analog Trigger Source (system)"=21951, "DAQmx Device Name (block diagram constant)"=2093, "DAQmx Device Name (classic)"=3318, "DAQmx Device Name (modern)"=21773, "DAQmx Device Name (system)"=21950, "DAQmx Global Channel (block diagram constant)"=3430, "DAQmx Global Channel (classic)"=3443, "DAQmx Global Channel (modern)"=21770, "DAQmx Global Channel (system)"=21957, "DAQmx Physical Channel (block diagram constant)"=2118, "DAQmx Physical Channel (classic)"=3335, "DAQmx Physical Channel (modern)"=21777, "DAQmx Physical Channel (system)"=21954, "DAQmx Scale Name (block diagram constant)"=2116, "DAQmx Scale Name (classic)"=3317, "DAQmx Scale Name (modern)"=21775, "DAQmx Scale Name (system)"=21952, "DAQmx Switch (block diagram constant)"=2121, "DAQmx Switch (classic)"=3337, "DAQmx Switch (modern)"=21776, "DAQmx Switch (system)"=21953, "DAQmx Task Name (block diagram constant)"=3434, "DAQmx Task Name (classic)"=3442, "DAQmx Task Name (modern)"=21778, "DAQmx Task Name (system)"=21959, "DAQmx Terminal (block diagram constant)"=2117, "DAQmx Terminal (classic)"=3319, "DAQmx Terminal (modern)"=21781, "DAQmx Terminal (system)"=21955, "Data Cache Size"=24132, "Data Log File Refnum"=3402, "Data Value Reference"=3476, "Data Value Reference Constant"=24134, "DataSocket Close"=1085, "DataSocket Open"=1084, "DataSocket Read"=1086, "DataSocket Refnum"=3417, "DataSocket Write"=1087, "Date/Time To Seconds"=1308, "Decimal Digit?"=1119, "Decimal String To Number"=1184, "Decimate 1D Array"=2046, "DecomposeArray"=2412, "DecomposeLockDataValRef"=2406, "DecomposeVariant"=2404, "Decrement"=1058, "Default Directory"=1427, "Delete"=8056, "Delete (deprecated)"=1417, "Delete Data Value Reference"=2409, "Delete From Array"=3912, "Delete Menu Items"=9004, "Delete Variant Attribute"=8206, "Delete Waveform Attribute"=8209, "Deny Access"=8057, "Dequeue Element"=9113, "Destroy Stream Endpoint"=23794, "Destroy User Event"=2075, "DevClear"=1961, "DevClearList"=1962, "Device Control/Status"=1433, "Device Refnum"=3405, "Diagram Disable Structure"=2054, "Dial (classic)"=3050, "Dial (modern)"=21732, "Digital Data (classic)"=3210, "Digital Data (modern)"=21216, "Digital Waveform Graph (classic)"=3511, "Digital Waveform Graph (modern)"=21718, "Direct Variable Read"=23785, "Direct Variable Write"=23788, "Divide"=1053, "Divide (with error terminals)"=3918, "Dlg Horiz Scrollbar"=21905, "Dlg Numeric #1"=2100, "Dlg Numeric #2"=3006, "Dlg String"=2110, "Dlg Vert Scrollbar"=21906, "Down Arrow"=3824, "Down Bow Valve (flat)"=3707, "Down Bow Valve (outline)"=3807, "Down Bow Valve (shaded)"=21767, "Down Rect Valve (flat)"=3706, "Down Rect Valve (outline)"=3806, "Down Rect Valve (shaded)"=21766, "Down Tee (flat)"=3818, "Down Tee (shaded)"=3718, "Dynamic FPGA Interface Cast"=5690, "Elementary Charge (C)"=23517, "Empty Array?"=23063, "Empty Path Constant"=23523, "Empty String Constant"=23503, "Empty String/Path?"=1112, "Enable Menu Tracking"=9002, "EnableLocal"=1963, "EnableRemote"=1964, "End of Line Constant"=23525, "Enqueue Element"=9111, "Enqueue Element At Opposite End"=9129, "Enum (classic)"=3023, "Enum (modern)"=21605, "Enum (system)"=3062, "Enum Constant"=2090, "EOF"=1410, "Equal To 0?"=1113, "Equal?"=1102, "Error Ring Constant"=2039, "Event Callback Refnum"=3435, "Event Data Node"=2102, "Event Structure"=2052, "Exchanger"=3828, "Exclusive Or"=1063, "Exponential"=1211, "Exponential (Arg) -1"=1222, "Expression Node"=2201, "False Constant"=2006, "Feedback Node"=2353, "FieldPoint IO Point (block diagram constant)"=3440, "FieldPoint IO Point (classic)"=3439, "FieldPoint IO Point (modern)"=21784, "FIFO Refnum"=3474, "File Dialog"=8058, "File Dialog (deprecated)"=8081, "File Path Control (classic)"=3203, "File Path Control (modern)"=21730, "File Path Control (system)"=21922, "File Path Indicator (classic)"=3204, "File Path Indicator (modern)"=21731, "File/Directory Info"=8082, "File/Directory Info (deprecated)"=1413, "FindLstn"=1965, "FindRQS"=1966, "First Call?"=1083, "Fixed-Point Overflow?"=5565, "Fixed-Point to Integer Cast"=5566, "Flat Box"=3602, "Flat Circle"=3605, "Flat Down Triangle"=3623, "Flat Frame"=3608, "Flat Left Triangle"=3620, "Flat Right Triangle"=3621, "Flat Round Button"=3102, "Flat Rounded Box"=3611, "Flat Sequence Structure"=2069, "Flat Square Button"=3103, "Flat Up Triangle"=3622, "Flatten To String"=1164, "Flatten To XML"=8400, "Flattened String To Variant"=8202, "Floating Point Equal?"=23064, "Flush File"=8059, "Flush File (deprecated)"=1406, "Flush Queue"=9114, "Flush Stream"=23808, "For Loop"=2002, "Fork"=2194, "Format Date/Time String"=8100, "Format Into File"=2083, "Format Into String"=2081, "Format Value"=1512, "Formula Node"=2004, "FPGA Refnum to Session"=2322, "Fract/Exp String To Number"=1187, "Framed Color Box (classic)"=3008, "Framed Color Box (modern)"=21019, "Free Label"=2321, "Furnace"=3829, "Gauge (classic)"=3040, "Gauge (modern)"=21009, "Gauge for Simon"=32600, "Generate Front Panel Activity"=1329, "Generate Occurrence"=1700, "Generate User Event"=2074, "Generate User-Defined Trace Event"=2250, "Get Datalog Position"=8061, "Get Date/Time In Seconds"=1303, "Get Date/Time String"=1600, "Get Drag Drop Data"=9154, "Get File Position"=8062, "Get File Size"=8063, "Get Fixed-Point Components"=11163, "Get Help Window Status"=1354, "Get Matrix Diagonal"=8501, "Get Matrix Elements"=8502, "Get Menu Item Info"=9005, "Get Menu Selection"=9001, "Get Menu Short Cut Info"=9007, "Get Notifier Status"=9103, "Get Number of Records"=8064, "Get Permissions"=8065, "Get Queue Status"=9110, "Get Submatrix"=8503, "Get Type and Creator"=8066, "Get Variant Attribute"=8205, "Get Volume Info"=8067, "Get Waveform Attribute"=8208, "Get Waveform Components"=2067, "Global Variable"=2060, "GPIB Clear"=1954, "GPIB Initialization"=1957, "GPIB Misc"=1956, "GPIB Read"=1951, "GPIB Serial Poll"=1955, "GPIB Status"=1959, "GPIB Trigger"=1953, "GPIB Wait"=1958, "GPIB Write"=1950, "Gravitational Constant (N m2/kg2)"=23519, "Greater Or Equal To 0?"=1114, "Greater Or Equal?"=1103, "Greater Than 0?"=1117, "Greater?"=1110, "Handle Peek"=1604, "Handle Poke"=1605, "Hex Digit?"=1123, "Hexadecimal String To Number"=1185, "Hopper #1"=21754, "Hopper #2"=3072, "Horiz Line"=3821, "Horiz Pipe (flat)"=3810, "Horiz Pipe (shaded)"=3710, "Horizontal Button Box"=3636, "Horizontal Fill Slide (classic)"=3012, "Horizontal Fill Slide (modern)"=21100, "Horizontal Gradient Oval"=32502, "Horizontal Gradient Rectangle"=32504, "Horizontal Gradient Rounded Rectangle"=32507, "Horizontal Graduated Bar"=21106, "Horizontal Pointer Slide (classic)"=3011, "Horizontal Pointer Slide (modern)"=21101, "Horizontal Pointer Slide (system)"=21902, "Horizontal Progress Bar (modern)"=21102, "Horizontal Progress Bar (system)"=21910, "Horizontal Scrollbar"=21110, "Horizontal Slide (classic)"=3010, "Horizontal Slide (system)"=21904, "Horizontal Slide Switch"=3114, "Horizontal Smooth Box"=3633, "Horizontal Splitter Bar"=21861, "Horizontal Splitter Bar (Classic)"=21863, "Horizontal Splitter Bar (System)"=21865, "Horizontal Switch"=3108, "Horizontal Tank"=3071, "Horizontal Toggle Switch (classic)"=3110, "Horizontal Toggle Switch (modern)"=21700, "Hyperbolic Cosecant"=23053, "Hyperbolic Cosine"=1215, "Hyperbolic Cotangent"=23055, "Hyperbolic Secant"=23054, "Hyperbolic Sine"=1214, "Hyperbolic Tangent"=1216, "IMAQ Session"=3415, "Implies"=1080, "In Place Element Structure"=2360, "In Range and Coerce"=1127, "Include Fixed-Point Overflow Status"=5564, "Increment"=1057, "Index & Bundle Cluster Array"=2056, "Index Array"=2042, "Index String Array"=1531, "Initialize Array"=2053, "Inline C Node"=2104, "Insert Into Array"=3911, "Insert Menu Items"=9003, "Integer to Fixed-Point Cast"=5567, "Intensity Chart (classic)"=3509, "Intensity Chart (modern)"=21719, "Intensity Graph (classic)"=3510, "Intensity Graph (modern)"=21720, "Interleave 1D Arrays"=2045, "Interpolate 1D Array"=1905, "Inverse Cosecant"=23050, "Inverse Cosine"=1207, "Inverse Cotangent"=23052, "Inverse Hyperbolic Cosecant"=23056, "Inverse Hyperbolic Cosine"=1218, "Inverse Hyperbolic Cotangent"=23058, "Inverse Hyperbolic Secant"=23057, "Inverse Hyperbolic Sine"=1217, "Inverse Hyperbolic Tangent"=1219, "Inverse Secant"=23051, "Inverse Sine"=1206, "Inverse Tangent"=1208, "Inverse Tangent (2 Input)"=1228, "Invoke Node"=3900, "IP To String"=1710, "IrDA Close Connection"=9144, "IrDA Create Listener"=9140, "IrDA Discover"=9141, "IrDA Network Connection Refnum"=3450, "IrDA Open Connection"=9142, "IrDA Read"=9145, "IrDA Wait On Listener"=9143, "IrDA Write"=9146, "IVI Delete Session"=8103, "IVI Logical Name (block diagram constant)"=3420, "IVI Logical Name (classic)"=3414, "IVI Logical Name (modern)"=21736, "IVI New Session"=8102, "Join"=2195, "Join Numbers"=1171, "Junction"=2197, "Knob (classic)"=3005, "Knob (modern)"=21000, "Label (modern)"=21960, "Label (system)"=21961, "Labeled Oblong Button"=3125, "Labeled Rectangular Button"=3124, "Labeled Round Button"=3122, "Labeled Square Button"=3123, "LabVIEW Object"=3457, "Leak Variant Value Reference"=2410, "LED Button"=3116, "Left Arrow"=3826, "Left Bow Valve (flat)"=3701, "Left Bow Valve (outline)"=3801, "Left Bow Valve (shaded)"=21761, "Left Down Elbow (flat)"=3811, "Left Down Elbow (shaded)"=3711, "Left Pump (flat)"=3813, "Left Pump (shaded)"=3713, "Left Rect Valve (flat)"=3700, "Left Rect Valve (outline)"=3800, "Left Rect Valve (shaded)"=21760, "Left Tee (flat)"=3809, "Left Tee (shaded)"=3709, "Left Up Elbow (flat)"=3808, "Left Up Elbow (shaded)"=3708, "Less Or Equal To 0?"=1115, "Less Or Equal?"=1104, "Less Than 0?"=1118, "Less?"=1111, "Lexical Class"=1126, "Line (chiseled, system)"=3632, "Line (chiseled, thick)"=3630, "Line (chiseled, thin)"=3627, "Line (thick)"=3629, "Line (thin)"=3626, "Line Feed Constant"=23501, "Line with Arrow (thick)"=3631, "Line with Arrow (thin)"=3628, "List Directory"=1418, "List Folder"=8083, "Listbox (classic)"=21806, "Listbox (modern)"=21792, "Listbox (system)"=21805, "Listbox Symbol Ring Constant"=2038, "Local Variable"=2061, "Lock Range"=1411, "Logarithm Base 10"=1210, "Logarithm Base 2"=1225, "Logarithm Base X"=1224, "Logical Shift"=1081, "Lossy Enqueue Element"=9130, "Lowered Box (thick)"=3635, "Lowered Rounded Box"=3638, "Machine Epsilon"=23528, "MakeAddr"=1967, "Mantissa & Exponent"=1150, "Match First String"=1532, "Match Pattern"=1535, "Match True/False String"=1533, "MathScript Call By Reference"=3906, "MathScript Node"=2357, "MATLAB script"=9020, "Matrix Size"=8507, "Max & Min"=1108, "Menu Refnum"=3413, "Menu Ring (classic)"=3018, "Menu Ring (modern)"=21600, "Menu-Popup Ring"=3017, "Merge Errors"=2147, "Merge Signals"=2350, "Meter (classic)"=3030, "Meter (modern)"=21008, "Mixed Checkbox (system)"=21333, "Mixed Signal Graph"=21721, "Molar Gas Constant (J/(mol K))"=23522, "Motion Resource (block diagram constant)"=3449, "Motion Resource (classic)"=3448, "Motion Resource (modern)"=21787, "Motor (flat)"=3820, "Motor (shaded)"=3720, "Move"=8068, "Move (deprecated)"=1415, "Multi-Segment Pipe"=23780, "Multicolumn Listbox (classic)"=21799, "Multicolumn Listbox (modern)"=21791, "Multicolumn Listbox (system)"=21798, "Multiply"=1052, "Multiply (with error terminals)"=3917, "Multiply Array Elements"=1904, "Multirate Structure"=2199, "Natural Logarithm"=1209, "Natural Logarithm (Arg +1)"=1221, "Natural Logarithm Base"=23510, "Natural Logarithm Of 10"=23513, "Natural Logarithm Of 2"=23514, "Natural Logarithm Of Pi"=23508, "Negate"=1069, "Negative Infinity"=23509, "New Data Value Reference"=2408, "New Directory"=1402, "New File"=1404, "New VI"=8014, "New VI Object"=8015, "Not"=1064, "Not A Number/Path/Refnum?"=1128, "Not A Path Constant"=23524, "Not a Refnum Constant"=23526, "Not a Shared Variable"=23527, "Not And"=1071, "Not Equal To 0?"=1116, "Not Equal?"=1105, "Not Exclusive Or"=1073, "Not Or"=1072, "Notifier Refnum"=3423, "Number of Cache Levels"=24133, "Number To Boolean Array"=1814, "Number To Decimal String"=1180, "Number To Engineering String"=1183, "Number To Exponential String"=1505, "Number To Fractional String"=1506, "Number To Hexadecimal String"=1181, "Number To Octal String"=1182, "Numeric Constant"=2005, "Numeric Control (classic)"=3000, "Numeric Control (modern)"=21003, "Numeric Control (system)"=21919, "Numeric Indicator (classic)"=3001, "Numeric Indicator (modern)"=21004, "Obtain Notifier"=9101, "Obtain Queue"=9108, "Occurrence Refnum"=3406, "Octal Digit?"=1129, "Octal String To Number"=1186, "OK Button (modern)"=21738, "OK Button (system)"=3130, "Old VISA Open"=1921, "OLE Variant"=3150, "One Button Dialog"=1340, "Open and Verify Variable Connection"=23790, "Open Application Reference"=8012, "Open Device"=1430, "Open File"=1403, "Open Tank (flat classic)"=21752, "Open Tank (shaded classic)"=3074, "Open Variable Connection"=23779, "Open Variable Connection in Background"=23791, "Open VI Object Reference"=8013, "Open VI Reference"=8010, "Open/Create/Replace Datalog"=8054, "Open/Create/Replace File"=8050, "Or"=1062, "Or Array Elements"=1910, "Oval with Shadow"=32509, "Package Matrix"=23001, "PassControl"=1968, "Path Constant"=2009, "Path to Array of Strings"=1423, "Path To String"=1077, "Path Type"=1421, "Pi"=23504, "Pi Divided By 2"=23506, "Pi Multiplied By 2"=23505, "Pick Line"=1510, "Pict Ring (classic)"=3015, "Pict Ring (modern)"=21602, "Pict Ring (system)"=21925, "PixMap"=3505, "PixMap (warning: dangerous)"=3507, "Planck's Constant (J/Hz)"=23516, "Platform Flat Square Button"=3134, "Plug-In Control"=21820, "Polar To Complex"=1047, "Polar To Re/Im"=23061, "Positive Infinity"=23515, "Power Of 10"=1212, "Power Of 2"=1223, "Power Of X"=1213, "PPoll"=1969, "PPollConfig"=1970, "PPollUnconfig"=1971, "Preallocated Read from Binary File"=24135, "Preserve Run-Time Class"=8018, "Pressure Tank (flat)"=3075, "Pressure Tank (shaded)"=21753, "Preview Queue Element"=9112, "Printable?"=1124, "Property Node"=1920, "Pulldown Menu Ring"=3061, "Push Button"=21001, "Queue Refnum"=3424, "Quit LabVIEW"=1352, "Quotient & Remainder"=1056, "Radio Button (system)"=3133, "Radio Buttons (classic)"=22003, "Radio Buttons (modern)"=22001, "Radio Buttons (system)"=22002, "Raised Box (classic)"=3600, "Raised Box (modern)"=3637, "Raised Circle"=3603, "Raised Down Triangle"=3615, "Raised Frame"=3606, "Raised Left Triangle"=3612, "Raised Right Triangle"=3613, "Raised Rounded Box"=3609, "Raised Up Triangle"=3614, "Random Number (0-1)"=1070, "RcvRespMsg"=1972, "Re/Im To Complex"=1046, "Re/Im To Polar"=23060, "Read Datalog"=8069, "Read Device"=1432, "Read File"=1407, "Read from Binary File"=8051, "Read from Text File"=8070, "Read Multiple Elements from Stream"=23803, "Read Single Element from Stream"=23797, "Read Variable"=23781, "Read Variable with Timeout"=23786, "ReadStatus"=1973, "Receive"=1974, "ReceiveSetup"=1975, "Recessed Box"=3601, "Recessed Circle"=3604, "Recessed Down Triangle"=3619, "Recessed Frame (modern)"=3607, "Recessed Frame (system)"=3624, "Recessed Left Triangle"=3616, "Recessed Menu Ring"=3019, "Recessed Right Triangle"=3617, "Recessed Rounded Box"=3610, "Recessed Up Triangle"=3618, "Reciprocal"=1059, "Reciprocal Of e"=23511, "Reciprocal Of Pi"=23507, "RecomposeArray"=2403, "RecomposeUnlockDataValRef (warning: dangerous)"=2407, "RecomposeVariant (warning: dangerous)"=2405, "Rectangular Stop Button"=3128, "Refnum to Path"=1424, "Refnum to Session"=2306, "Region"=2196, "Register Event Callback"=2078, "Register For Events"=2065, "Register Session"=2319, "Release Notifier"=9102, "Release Queue"=9109, "Remove Fixed-Point Overflow Status"=5563, "Replace Array Subset"=3910, "Replace Substring"=3913, "Request Deallocation"=1610, "ResetSys"=1976, "Reshape Array"=2055, "Resize Matrix"=8508, "Resource Index"=1088, "Reverse 1D Array"=1900, "Reverse String"=1537, "Right Arrow"=3825, "Right Bow Valve (flat)"=3705, "Right Bow Valve (outline)"=3805, "Right Bow Valve (shaded)"=21765, "Right Down Elbow (flat)"=3817, "Right Down Elbow (shaded)"=3717, "Right Pump (flat)"=3819, "Right Pump (shaded)"=3719, "Right Rect Valve (flat)"=3704, "Right Rect Valve (outline)"=3804, "Right Rect Valve (shaded)"=21764, "Right Tee (flat)"=3815, "Right Tee (shaded)"=3715, "Right Up Elbow (flat)"=3814, "Right Up Elbow (shaded)"=3714, "Rocker"=21002, "Rotary Feeder"=3830, "Rotate"=1082, "Rotate 1D Array"=1906, "Rotate Left With Carry"=1606, "Rotate Right With Carry"=1607, "Rotate String"=1536, "Round Button"=3100, "Round LED (classic)"=3120, "Round LED (modern)"=21012, "Round Light"=3104, "Round Push Button"=3118, "Round Push Button (profile)"=3112, "Round Radio Button"=3106, "Round Stop Button"=3127, "Round To Nearest"=1055, "Round Toward +Infinity"=1076, "Round Toward -Infinity"=1075, "Rounded Rectangle with Shadow"=32508, "RT FIFO Create"=24000, "RT FIFO Delete"=24003, "RT FIFO Read"=24001, "RT FIFO Write"=24002, "Rydberg Constant (1/m)"=23521, "Scale By Power Of 2"=1074, "Scan From File"=2082, "Scan From String"=2080, "Scan String For Tokens"=8101, "Scan Value"=1534, "Scanned Variable Read"=23784, "Scanned Variable Write"=23787, "Search 1D Array"=1901, "Search and Replace String"=3914, "Search Variable Container"=23802, "Search/Split String"=1538, "Secant"=1203, "Seconds To Date/Time"=1309, "Seek"=1409, "Select"=1516, "Send"=1977, "Send Notification"=9104, "SendCmds"=1978, "SendDataBytes"=1979, "SendIFC"=1980, "SendList"=1981, "SendLLO"=1982, "SendSetup"=1983, "Session to Refnum"=2307, "Set Datalog Position"=8072, "Set File Position"=8073, "Set File Size"=8074, "Set Matrix Diagonal"=8504, "Set Matrix Elements"=8505, "Set Menu Item Info"=9006, "Set Number of Records"=8075, "Set Occurrence"=1702, "Set Permissions"=8076, "Set Submatrix"=8506, "Set Type and Creator"=8077, "Set Variant Attribute"=8204, "Set Waveform Attribute"=8207, "SetRWLS"=1984, "SetTimeOut"=1985, "Shared Variable"=23778, "Shared Variable Constant"=3473, "Shared Variable Control (classic)"=3472, "Shared Variable Control (modern)"=21814, "Shared Variable to String"=1831, "Sign"=1049, "Simple Horizontal Slide"=3003, "Simple Numeric"=2900, "Simple String"=2115, "Simple Vertical Slide"=3002, "Sinc"=1227, "Sine"=1200, "Sine & Cosine"=1220, "Size Handle"=1603, "Slide Switch"=21011, "Smoothed Oval"=32500, "Smoothed Rounded Rectangle"=32505, "Sort 1D Array"=1120, "Sort Array of String"=23065, "Speed Of Light In Vacuum (m/sec)"=23518, "Spin Control (system)"=21900, "Split 1D Array"=1908, "Split Button"=21020, "Split Number"=1170, "Split Signals"=2351, "Spreadsheet String To Array"=1539, "Square"=23059, "Square Button"=3101, "Square LED (classic)"=3121, "Square LED (modern)"=21013, "Square Light"=3105, "Square Push Button"=3119, "Square Push Button (profile)"=3113, "Square Radio Button"=3107, "Square Root"=1060, "Stacked Sequence Structure"=2000, "State"=2198, "State Diagram"=2051, "Static VI Reference"=2084, "Stop"=1350, "Stop Button"=21230, "String Constant"=2007, "String Control (classic)"=3200, "String Control (modern)"=21701, "String Control (system)"=21920, "String Indicator (classic)"=3201, "String Indicator (modern)"=21702, "String Length"=1502, "String Subset"=1503, "String To Byte Array"=1608, "String To IP"=1711, "String To Path"=1078, "String to Shared Variable"=1830, "Strip Path"=1420, "SubPanel"=21810, "SubPanel (Classic)"=21811, "SubPanel (System)"=21823, "Subtract"=1051, "Subtract (with error terminals)"=3916, "Swap Bytes"=1162, "Swap Values"=2401, "Swap Vector Element"=1912, "Swap Words"=1163, "Tab Constant"=23502, "Tab Control (classic)"=3330, "Tab Control (modern)"=3332, "Tab Control (system)"=3331, "Table (classic)"=21796, "Table (modern)"=21790, "Table (system)"=21797, "Tag Attribute Ring"=2063, "Tangent"=1202, "Tank (classic)"=3020, "Tank (modern)"=21006, "TCP Close Connection"=1713, "TCP Create Listener"=1717, "TCP Flattened Read"=1718, "TCP Flattened Write"=1719, "TCP Flex Read"=1720, "TCP Flex Write"=1721, "TCP Network Connection Refnum"=3407, "TCP Open Connection"=1715, "TCP Read"=1716, "TCP Wait On Listener"=1712, "TCP Write"=1714, "TDMS Close"=24113, "TDMS Defragment"=24119, "TDMS File"=3477, "TDMS Flush"=24117, "TDMS Get Properties"=24115, "TDMS List Contents"=24116, "TDMS Open"=24112, "TDMS Read"=24111, "TDMS Refnum To File ID"=24120, "TDMS Set Properties"=24114, "TDMS Write"=24110, "TDMS Write IP"=24118, "Temporary Directory"=1435, "TestSRQ"=1986, "TestSys"=1987, "Text & Pict Ring (classic)"=3016, "Text & Pict Ring (modern)"=21603, "Text Button"=21015, "Text Ring (block diagram constant)"=2008, "Text Ring (classic)"=3014, "Text Ring (modern)"=21601, "Text Ring (system)"=3060, "Text to UTF-8"=23066, "Thermometer (classic)"=3021, "Thermometer (modern)"=21007, "Threshold 1D Array"=1909, "Tick Count (ms)"=1300, "Time Stamp (block diagram constant)"=2068, "Time Stamp Control (classic)"=5555, "Time Stamp Control (modern)"=21913, "Time Stamp Control (system)"=21967, "Time Stamp Indicator (classic)"=5556, "Time Stamp Indicator (modern)"=21914, "Timed Loop"=5570, "Timed Sequence"=5573, "To Byte Integer"=1140, "To Double Precision Complex"=1152, "To Double Precision Float"=1147, "To Extended Precision Complex"=1154, "To Extended Precision Float"=1149, "To Fixed-Point"=5561, "To Long Integer"=1142, "To Lower Case"=1189, "To More Generic Class"=8017, "To More Specific Class"=8016, "To OLE Variant"=8002, "To Probe String"=2413, "To Quad Integer"=1155, "To Single Precision Complex"=1151, "To Single Precision Float"=1146, "To Time Stamp"=5560, "To Unsigned Byte Integer"=1143, "To Unsigned Long Integer"=1145, "To Unsigned Quad Integer"=1156, "To Unsigned Word Integer"=1144, "To Upper Case"=1188, "To Variant"=8201, "To Word Integer"=1141, "Traditional DAQ Channel (block diagram constant)"=2085, "Traditional DAQ Channel (classic)"=3320, "Traditional DAQ Channel (modern)"=21733, "Transpose 1D Array"=23068, "Transpose 2D Array"=1902, "Transpose Matrix"=8509, "Tree (classic)"=21819, "Tree (modern)"=21793, "Tree (system)"=21794, "Trigger"=1988, "TriggerList"=1989, "Two Button Dialog"=1341, "Type and Creator"=1434, "Type Cast"=1166, "UDP Close"=1726, "UDP Multicast Open"=1727, "UDP Network Connection Refnum"=3418, "UDP Open"=1723, "UDP Read"=1724, "UDP Write"=1725, "Unbitpack from Array"=3136, "Unbundle"=2048, "Unbundle By Name"=2058, "Unflatten From String"=1165, "Unflatten From XML"=8401, "Unleak Variant Value Reference"=2411, "Unpackage Matrix"=23000, "Unregister For Events"=2076, "Unregister Session"=2320, "Up Arrow"=3823, "Up Bow Valve (flat)"=3703, "Up Bow Valve (outline)"=3803, "Up Bow Valve (shaded)"=21763, "Up Rect Valve (flat)"=3702, "Up Rect Valve (outline)"=21762, "Up Rect Valve (shaded)"=3802, "Up Tee (flat)"=3812, "Up Tee (shaded)"=3712, "User Defined Refnum"=3428, "User Defined Refnum Tag (block diagram constant)"=3426, "User Defined Refnum Tag (classic)"=3429, "User Defined Refnum Tag (modern)"=21745, "User Defined Refnum Tag Flatten (classic)"=3454, "User Defined Refnum Tag Flatten (modern)"=21747, "User Defined Tag (block diagram constant)"=2114, "User Defined Tag (classic)"=3329, "User Defined Tag (modern)"=21749, "User Item"=3506, "UTF-8 to Text"=23067, "Variable Class Specifier Constant"=2106, "Variable Configuration"=3475, "Variable Name Constant"=3478, "Variant"=3310, "Variant To Data"=8003, "Variant To Flattened String"=8203, "Vert Line"=3822, "Vert Pipe (flat)"=3816, "Vert Pipe (shaded)"=3716, "Vert Rocker"=21740, "Vertical Fill Slide (classic)"=3009, "Vertical Fill Slide (modern)"=21014, "Vertical Gradient Oval"=32501, "Vertical Gradient Rectangle"=32503, "Vertical Gradient Rounded Rectangle"=32506, "Vertical Graduated Bar"=21107, "Vertical Pointer Slide (classic)"=3007, "Vertical Pointer Slide (modern)"=21017, "Vertical Pointer Slide (system)"=21901, "Vertical Progress Bar (modern)"=21104, "Vertical Progress Bar (system)"=21909, "Vertical Scrollbar"=21111, "Vertical Slide"=3004, "Vertical Slide (system)"=21903, "Vertical Slide Switch (classic)"=3115, "Vertical Slide Switch (modern)"=21741, "Vertical Smooth Box"=3634, "Vertical Splitter Bar"=21860, "Vertical Splitter Bar (Classic)"=21862, "Vertical Splitter Bar (System)"=21864, "Vertical Switch"=3109, "Vertical Toggle Switch (classic)"=3111, "Vertical Toggle Switch (modern)"=21005, "VI Library"=1425, "VI Refnum"=3422, "VI Server Reference"=2091, "VISA Assert Interrupt Signal"=2309, "VISA Assert Trigger"=1929, "VISA Assert Utility Signal"=2310, "VISA Clear"=1927, "VISA Close"=1922, "VISA Disable Event"=1940, "VISA Discard Events"=1941, "VISA Enable Event"=1942, "VISA Find Resource"=1923, "VISA Flush I/O Buffer"=2302, "VISA GPIB Command"=2315, "VISA GPIB Control ATN"=2316, "VISA GPIB Control REN"=2304, "VISA GPIB Pass Control"=2317, "VISA GPIB Send IFC"=2318, "VISA In 16"=1930, "VISA In 32"=1944, "VISA In 64"=2140, "VISA In 8"=1936, "VISA Lock"=1993, "VISA Map Address"=1932, "VISA Map Trigger"=2311, "VISA Memory Allocation"=1997, "VISA Memory Allocation Ex"=2146, "VISA Memory Free"=1998, "VISA Move"=2303, "VISA Move In 16"=1948, "VISA Move In 32"=1991, "VISA Move In 64"=2144, "VISA Move In 8"=1946, "VISA Move Out 16"=1949, "VISA Move Out 32"=1992, "VISA Move Out 64"=2145, "VISA Move Out 8"=1947, "VISA Open"=2308, "VISA Out 16"=1931, "VISA Out 32"=1945, "VISA Out 64"=2141, "VISA Out 8"=1937, "VISA Peek 16"=1934, "VISA Peek 32"=1995, "VISA Peek 64"=2142, "VISA Peek 8"=1938, "VISA Poke 16"=1935, "VISA Poke 32"=1996, "VISA Poke 64"=2143, "VISA Poke 8"=1939, "VISA Read"=1925, "VISA Read STB"=1928, "VISA Read To File"=2313, "VISA Refnum to Session"=2300, "VISA Resource Name"=3421, "VISA resource name (classic)"=3409, "VISA resource name (modern)"=21737, "VISA Set I/O Buffer Size"=2301, "VISA Status Description"=1924, "VISA Unlock"=1994, "VISA Unmap Address"=1933, "VISA Unmap Trigger"=2312, "VISA USB Control In"=2086, "VISA USB Control Out"=2087, "VISA VXI Cmd or Query"=2305, "VISA Wait on Event"=1943, "VISA Write"=1926, "VISA Write From File"=2314, "Volume Info"=1414, "Wait (ms)"=1302, "Wait For Activity"=1722, "Wait For Front Panel Activity"=1328, "Wait for GPIB RQS"=1952, "Wait on Notification"=9105, "Wait on Notification from Multiple"=9106, "Wait on Notification from Multiple with Notifier History"=9132, "Wait on Notification with Notifier History"=9131, "Wait on Occurrence"=1701, "Wait Until Next ms Multiple"=1327, "WaitSRQ"=1990, "Waveform Chart"=21010, "Waveform Chart (classic)"=3501, "Waveform Chart (modern)"=21717, "Waveform Graph (classic)"=3504, "Waveform Graph (modern)"=21703, "While Loop #1"=2003, "While Loop #2"=2352, "White Space?"=1125, "Write Datalog"=8079, "Write Device"=1431, "Write File"=1408, "Write Multiple Elements to Stream"=23804, "Write Single Element to Stream"=23798, "Write to Binary File"=8078, "Write to Text File"=8080, "Write Variable"=23782, "Write Variable with Timeout"=23789, "XY Graph (classic)"=3500, "XY Graph (modern)"=21716, "Y-th Root of X"=23062]
  n1 = New VI() -> (0:w15:errorcluster, 3:w16:refnum<vi>)  [unwired: 7 in]
  n2 = property class="VI"(reference=w16, error in=w15, "BDWin.Open"=TRUE ("Block Diagram Window:Open")) -> (reference out=w2:refnum<vi>, error out=w12:errorcluster, "Diagram"=w13:refnum<vi>)
  n3 = New VI Object(vi object class=w9, owner refnum=w13, style=w11, position/next to=T1 {"Horizontal"=10, "Vertical"=10} ("location"), 8:w12) -> (object refnum=w8:refnum<vi>, 0:w7:errorcluster)  [unwired: 3 in]
  n4 = invoke class="BoolCnst" method="Set Property"(reference=w8, error in=w7, "Index"=w5, "Value"="Colors [1]") -> (reference out=w4:refnum<vi>, error out=w3:errorcluster)  [unwired: 1 in, 3 out]
  n5 = invoke class="BoolCnst" method="ObjHighlight"(reference=w4, error in=w3) -> (error out=w1:errorcluster)  [unwired: 1 in, 2 out]
  n6 = Close Reference(reference=w2, error in (no error)=w1) -> ()  [unwired: 1 out]
